vi "RANGE Startup File.vi"(11 "appended path":path) -> (3 "new file path (Not A Path if cancelled)":path)   [LabVIEW 2023]
uses:
  Drivers/Omega FMA-1600A Series Gas Flow Meter/Type Definitions/FMA1600A Gas Type.ctl
  Drivers/Omega FMA-1600A Series Gas Flow Meter/Type Definitions/FMA1600A Meter Accuracy Options.ctl
  <vilib>/Utility/file.llb/Write To Spreadsheet File (string).vi
panel:
  in  "Disable All Meters":bool
  in  "Complete":bool
  in  "Meter Accuracy Option 6":T1
  in  "Gas Meter 6":T2
  in  "Meter Accuracy Option 5":T1
  in  "Gas Meter 5":T2
  in  "Meter Accuracy Option 4":T1
  in  "Gas Meter 4":T2
  in  "Meter Accuracy Option 3":T1
  in  "Gas Meter 3":T2
  in  "Meter Accuracy Option 2":T1
  in  "Gas Meter 2":T2
  in  "Meter Accuracy Option 1":T1
  in  "Gas Meter 1":T2
  in  "Update Gas Type":bool
  in  "Tab Control":enum32{"Page 1"}(tab)
  out "Start Up File 2":string[][](array[string])
  in  "Start Up File":string[][](array[string])
  # "+/- 0.8% RDG + 0.2% FS = Standard\n+/- 0.4% RDG + 0.2% FS = HCAL (Optional when Purchased)"
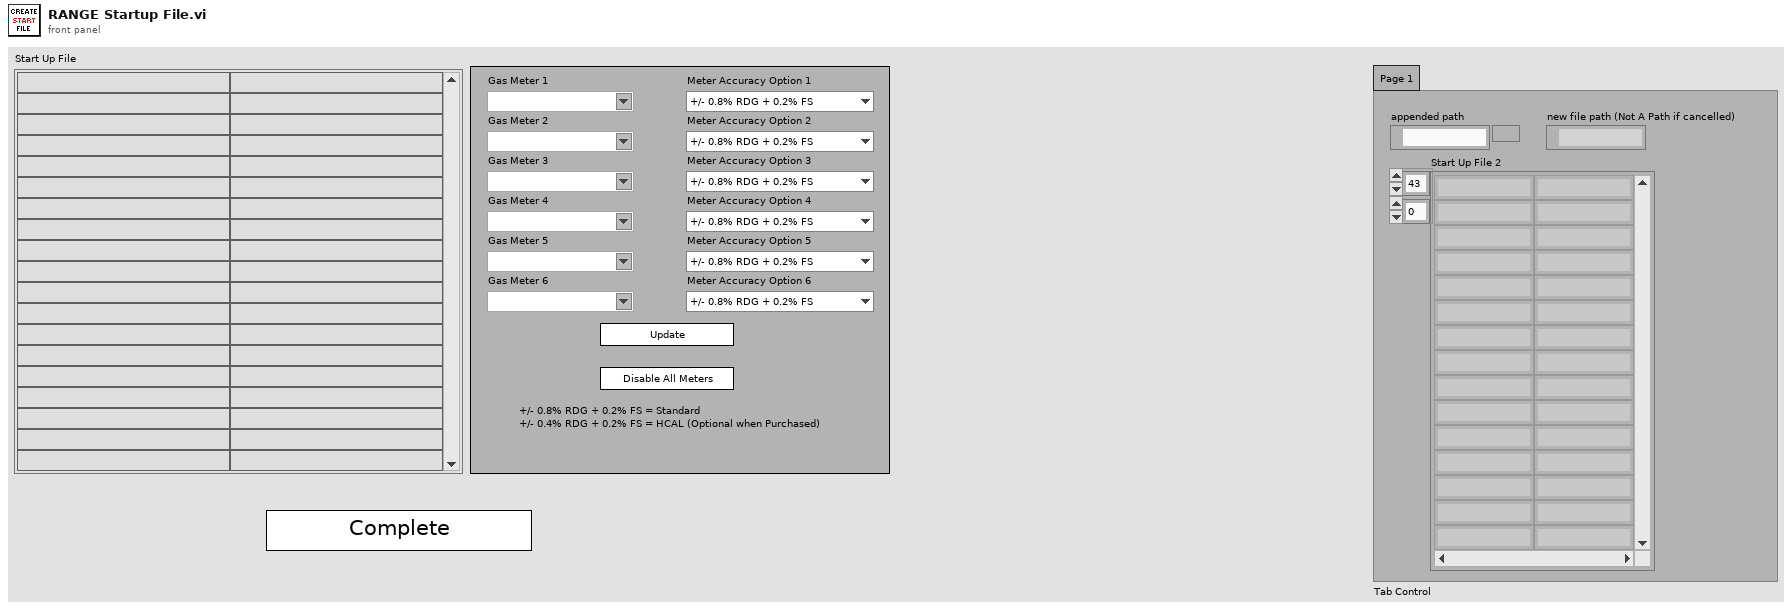
[diagram p1: front panel]
types:
  T1 = typedef "FMA1600A Meter Accuracy Options.ctl" = enum16{"+/- 0.8% RDG + 0.2% FS", "+/- 0.4% RDG + 0.2% FS"}
  T2 = typedef "FMA1600A Gas Type.ctl" = string
  T3 = enum32{"invalid app kind", "Development System", "Run Time System", "Student Edition", "Embedded LabVIEW", "Evaluation", "Custom"}
  T4 = enum32{"Invalid", "Standard", "Closed", "Hidden", "Minimized", "Maximized"}
  T5 = cluster{"Core":cluster{"Current VI Reference":refnum<vi>, "Close Panel on Exit?":bool}, "Start Up File":string[][]}
  T6 = cluster{"Current VI Reference":refnum<vi>, "Close Panel on Exit?":bool}
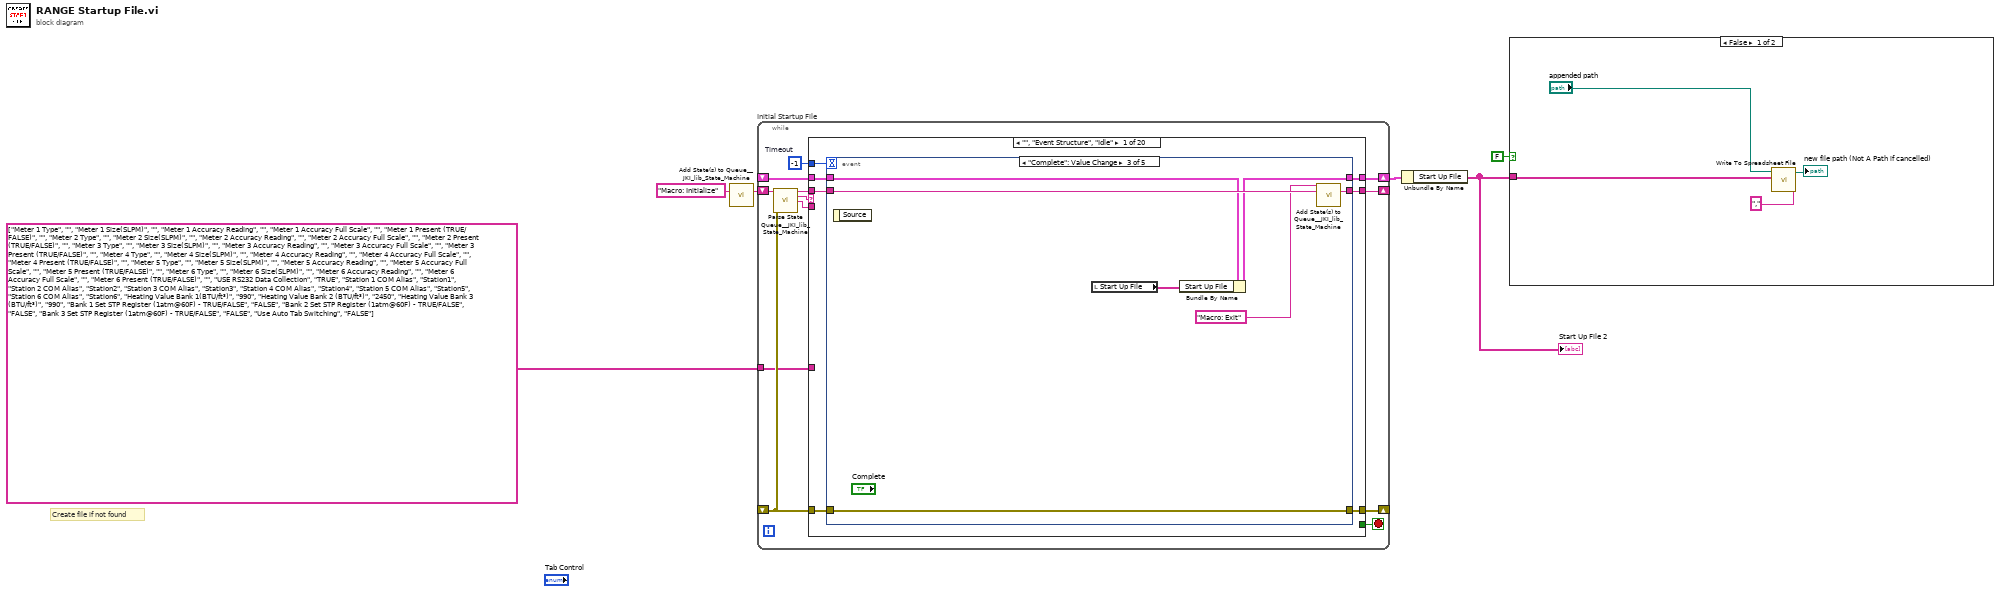
[diagram p0: block diagram]
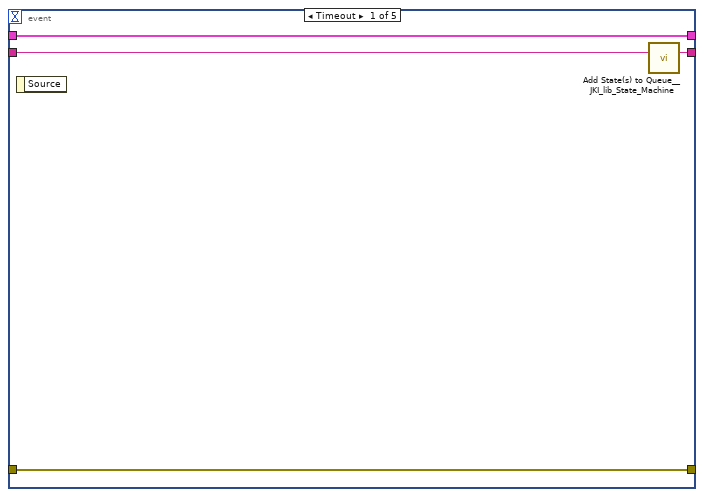
[diagram p2: hidden frame]
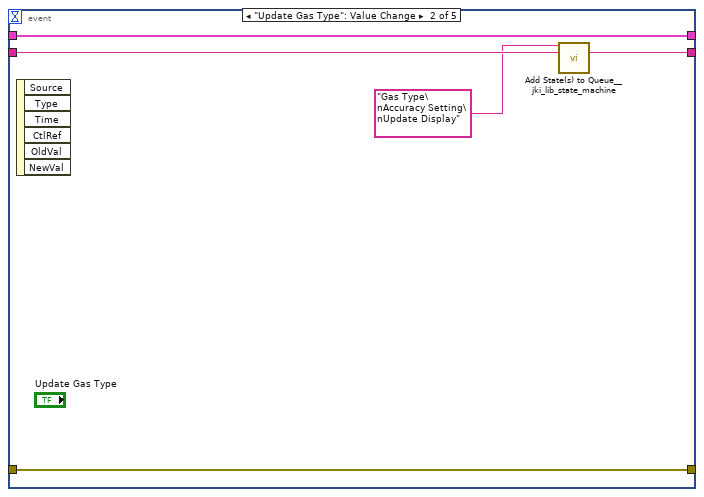
[diagram p3: hidden frame]
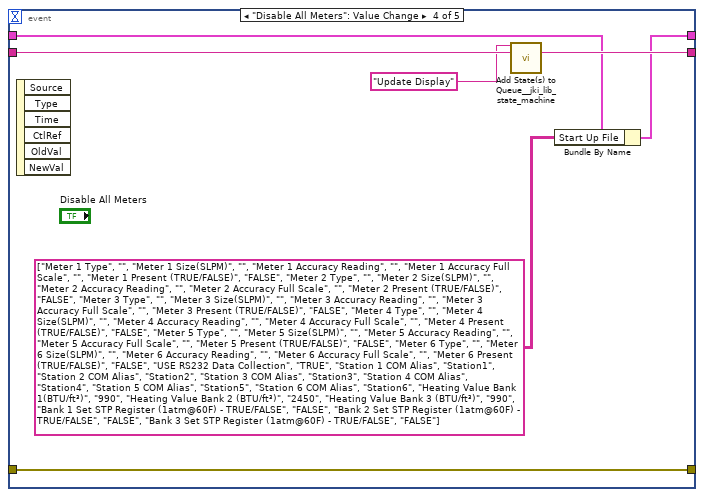
[diagram p4: hidden frame]
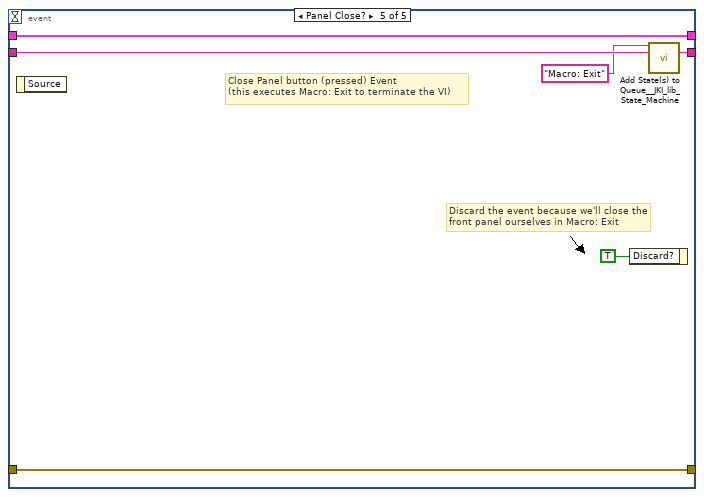
[diagram p5: hidden frame]
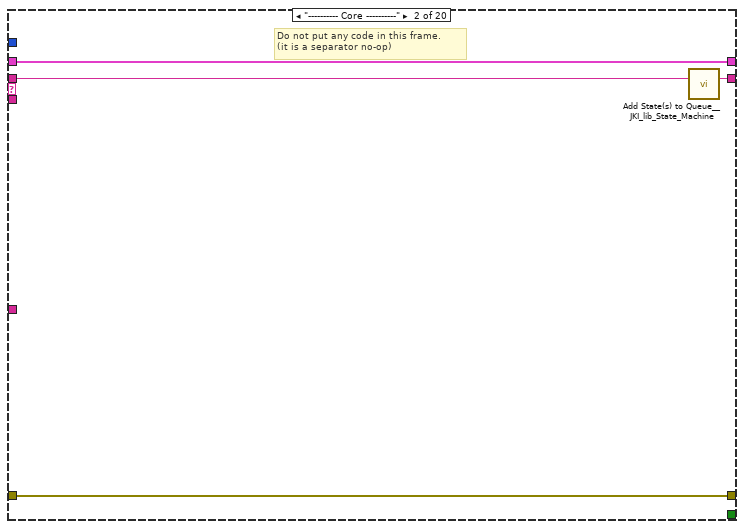
[diagram p6: hidden frame]
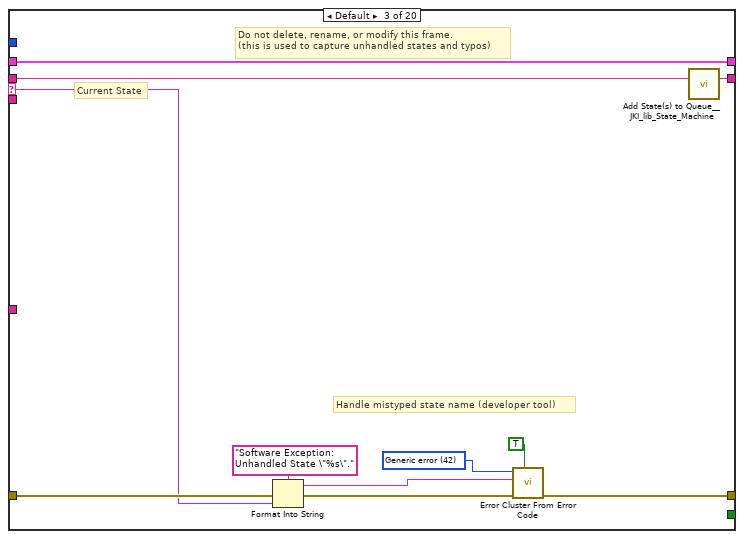
[diagram p7: hidden frame]
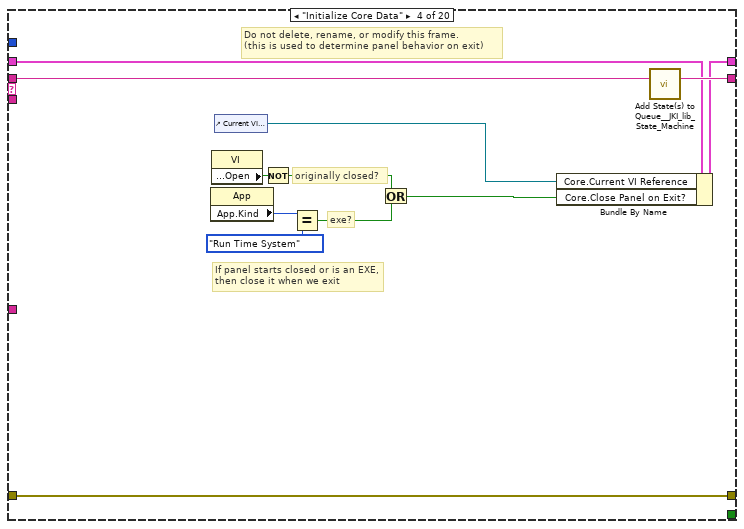
[diagram p8: hidden frame]
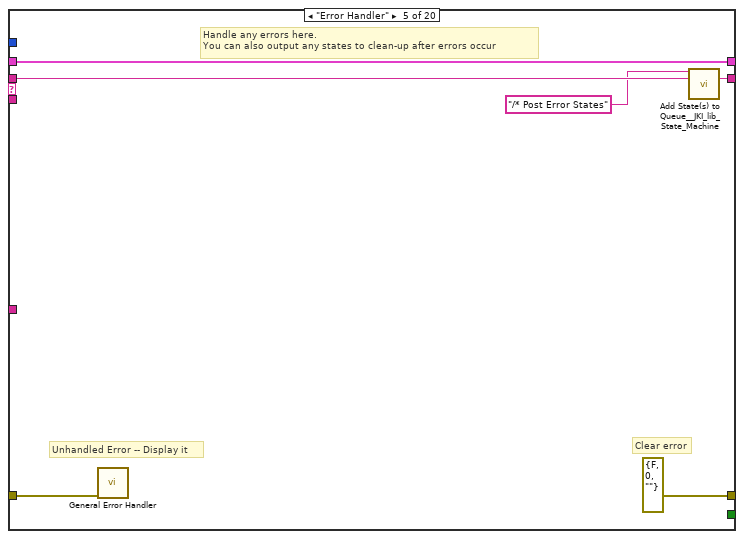
[diagram p9: hidden frame]
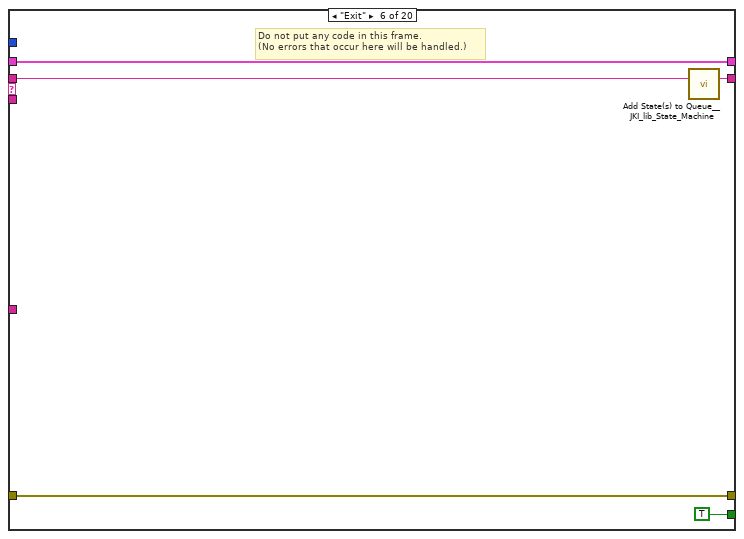
[diagram p10: hidden frame]
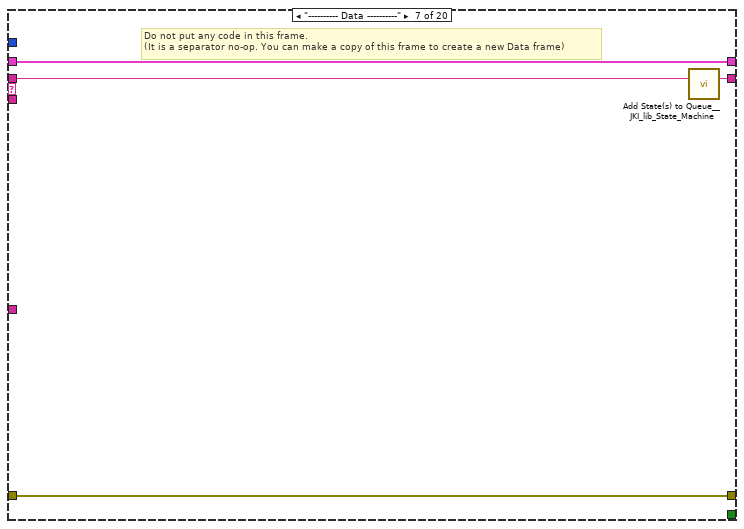
[diagram p11: hidden frame]
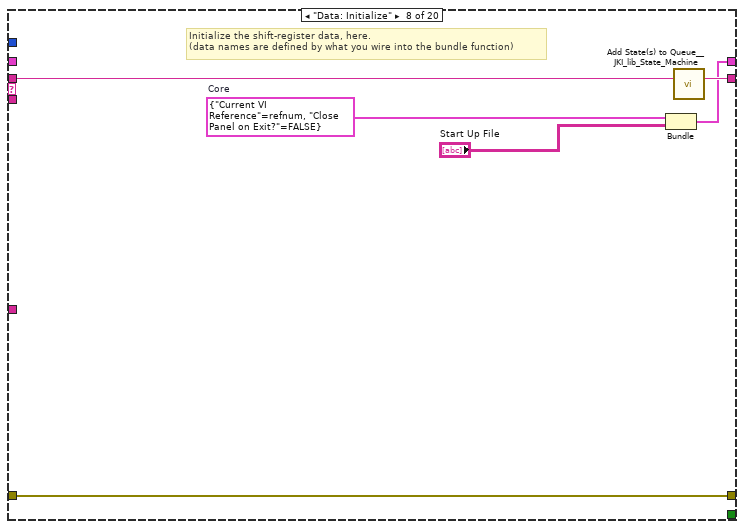
[diagram p12: hidden frame]
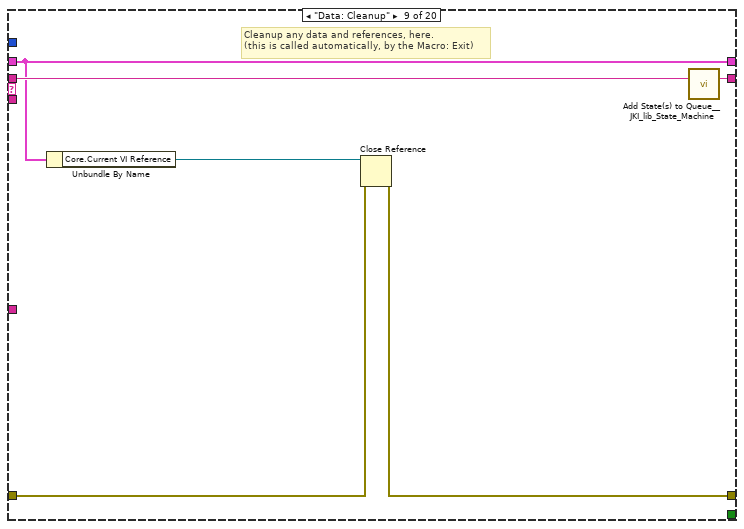
[diagram p13: hidden frame]
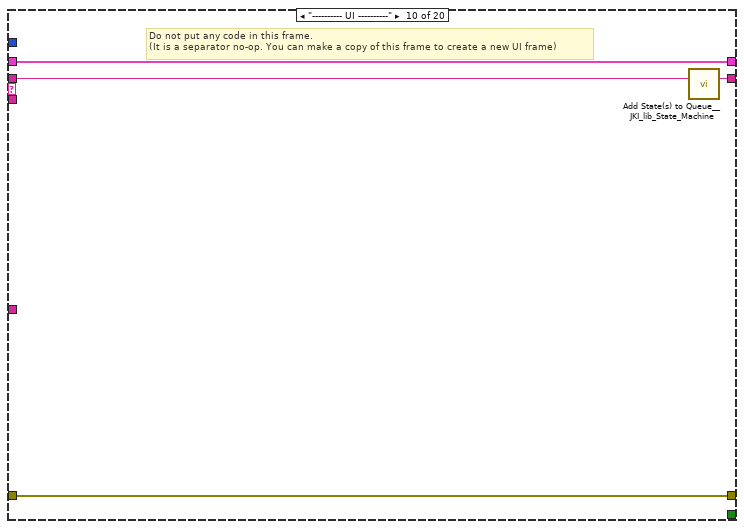
[diagram p14: hidden frame]
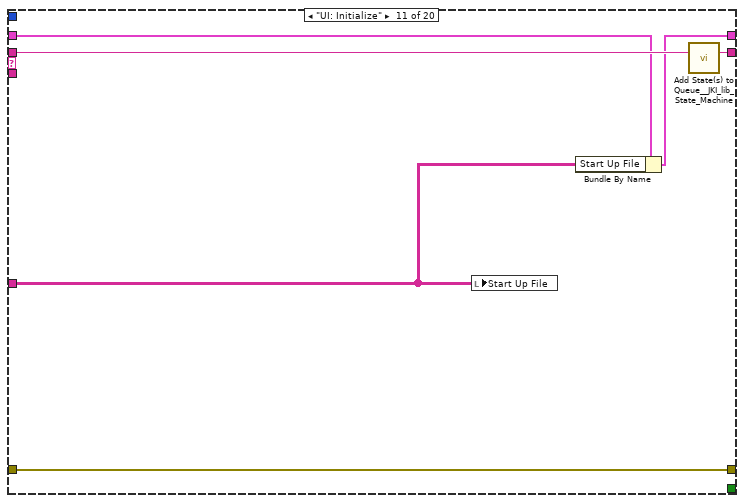
[diagram p15: hidden frame]
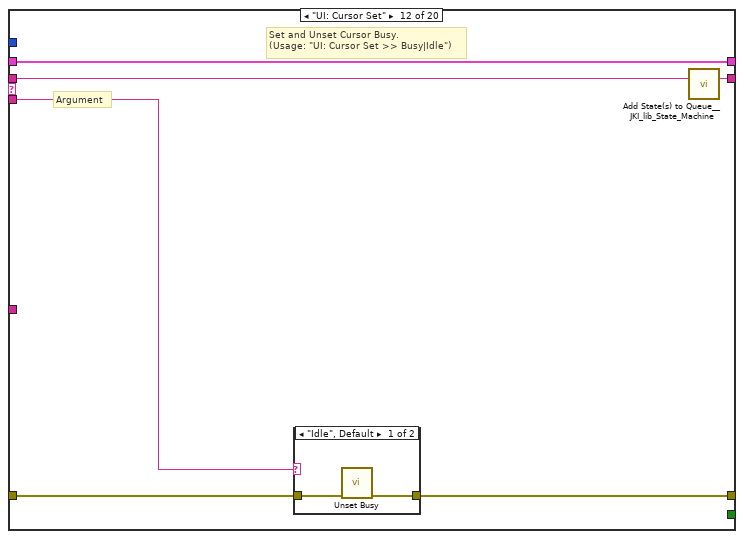
[diagram p16: hidden frame]
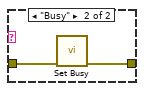
[diagram p17: hidden frame]
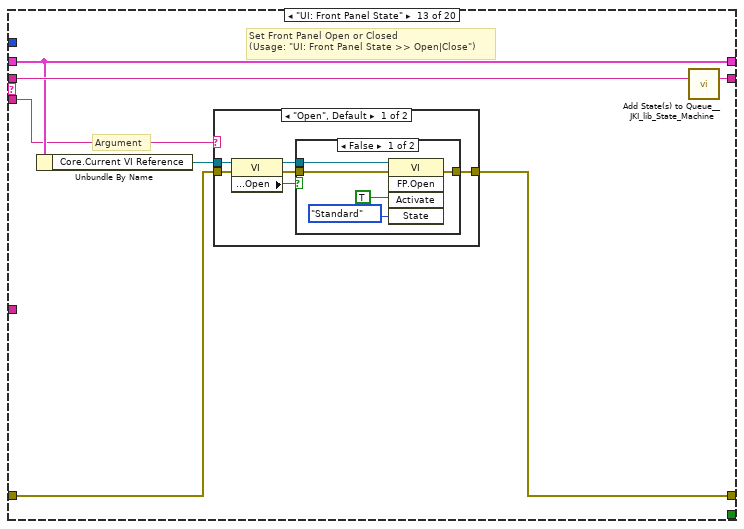
[diagram p18: hidden frame]
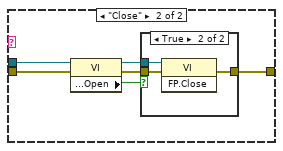
[diagram p20: hidden frame]
diagram:
  # "Create file if not found"
  n1 = call <vilib>:"Add State(s) to Queue__JKI_lib_State_Machine.vi"("State(s) in (\"\")"="Macro: Initialize") -> ("States Out"=w5:string)  [unwired: 14 in]
  n2 = while "Initial Startup File" {
    shift-right: [w11] -> w3
    shift-left: _ -> [w10]
    shift-right: [w14] -> _
    shift-left: _ -> [w8]
    shift-right: [w13] -> _
    shift-left: w5 -> [w15]
    tunnel: string[][] [["Meter 1 Type", ""], ["Meter 1 Size(SLPM)", ""], ["Meter 1 Accuracy Reading", ""], ["Meter 1 Accuracy Full Scale", ""], ["Meter 1 Present (TRUE/FALSE)", ""], ["Meter 2 Type", ""], ["Meter 2 Size(SLPM)", ""], ["Meter 2 Accuracy Reading", ""], ["Meter 2 Accuracy Full Scale", ""], ["Meter 2 Present (TRUE/FALSE)", ""], ["Meter 3 Type", ""], ["Meter 3 Size(SLPM)", ""], ["Meter 3 Accuracy Reading", ""], ["Meter 3 Accuracy Full Scale", ""], ["Meter 3 Present (TRUE/FALSE)", ""], ["Meter 4 Type", ""], ["Meter 4 Size(SLPM)", ""], ["Meter 4 Accuracy Reading", ""], ["Meter 4 Accuracy Full Scale", ""], ["Meter 4 Present (TRUE/FALSE)", ""], ["Meter 5 Type", ""], ["Meter 5 Size(SLPM)", ""], ["Meter 5 Accuracy Reading", ""], ["Meter 5 Accuracy Full Scale", ""], ["Meter 5 Present (TRUE/FALSE)", ""], ["Meter 6 Type", ""], ["Meter 6 Size(SLPM)", ""], ["Meter 6 Accuracy Reading", ""], ["Meter 6 Accuracy Full Scale", ""], ["Meter 6 Present (TRUE/FALSE)", ""], ["USE RS232 Data Collection", "TRUE"], ["Station 1 COM Alias", "Station1"], ["Station 2 COM Alias", "Station2"], ["Station 3 COM Alias", "Station3"], ["Station 4 COM Alias", "Station4"], ["Station 5 COM Alias", "Station5"], ["Station 6 COM Alias", "Station6"], ["Heating Value Bank 1(BTU/ft³)", "990"], ["Heating Value Bank 2 (BTU/ft³)", "2450"], ["Heating Value Bank 3 (BTU/ft³)", "990"], ["Bank 1 Set STP Register (1atm@60F) - TRUE/FALSE", "FALSE"], ["Bank 2 Set STP Register (1atm@60F) - TRUE/FALSE", "FALSE"], ["Bank 3 Set STP Register (1atm@60F) - TRUE/FALSE", "FALSE"], ["Use Auto Tab Switching", "FALSE"]] ("all rows 2") -> [w7]
    stop <- w12 stop-if-true
    w9 = -1  # Timeout
    n3 = call <vilib>:"Parse State Queue__JKI_lib_State_Machine.vi"("State Queue"=w15, "Error In (no error)"=w8) -> ("Remaining States"=w17:string, "Current State"=w18:string, "Arguments"=w16:string)  [unwired: 11 in]
    n4 = case shown="\"\", \"Event Structure\", \"Idle\"" w18 {
      selector: w18 -> [_ _ w59 _ _ _ _ _ _ _ _ _ _ _ _ _ _ _ _ _]
      tunnel: w17 -> [w25 w58 w63 w81 w87 w92 w96 w102 w108 w112 w118 w124 w135 w161 w166 w176 w180 w194 w208 w213]
      tunnel: w16 -> [_ _ _ _ _ _ _ _ _ _ _ w119 w129 _ _ _ _ _ _ _]
      tunnel: w10 -> [w23 w55 w61 w72 w84 w90 w93 _ w103 w109 w115 w122 w131 w158 w163 w173 w177 w192 w205 w210]
      tunnel: [w22 w56 w65 w78 errorcluster {"status"=FALSE, "code"=0, "source"=""} ("error out") w89 w94 w99 w104 w110 w116 w120 w132 w159 w164 w174 w178 w181 w201 w211] -> w14
      tunnel: w8 -> [w21 w56 w64 w78 w83 w89 w94 w99 w105 w110 w116 w121 w133 w159 w164 w174 w178 w182 w202 w211]
      tunnel: [w24 w57 w62 w80 w86 w91 w95 w101 w107 w111 w117 w123 w134 w160 w165 w175 w179 w193 w207 w212] -> w13
      tunnel: [_ _ _ _ _ TRUE _ _ _ _ _ _ _ _ _ _ _ _ _ _] -> w12
      tunnel: [w20 w55 w61 w79 w84 w90 w93 w100 w103 w109 w114 w122 w131 w158 w163 w173 w177 w191 w204 w210] -> w11
      tunnel: w9 -> [w19 _ _ _ _ _ _ _ _ _ _ _ _ _ _ _ _ _ _ _]
      tunnel: w7 -> [_ _ _ _ _ _ _ _ _ _ w113 _ _ _ _ _ _ _ _ _]
      frame "", "Event Structure", "Idle" {
        n5 = event shown="[2] \"Complete\": Value Change" {
          selector: _ -> [_ _ _ _ _]
          dyn-events: _ -> [_ _ _ _ _]
          timeout: w19 -> [_ _ _ _ _]
          tunnel: w25 -> [w29 w32 w41 w47 w54]
          tunnel: [w28 w31 w40 w46 w53] -> w24
          tunnel: w23 -> [w26 w33 w37 w44 w51]
          tunnel: [w27 w34 w39 w48 w52] -> w22
          tunnel: w21 -> [w27 w34 w39 w48 w52]
          tunnel: [w26 w33 w36 w43 w51] -> w20
          event Timeout {
            n6 = event-data() -> ()  [unwired: 1 in, 1 out]
            n7 = call <vilib>:"Add State(s) to Queue__JKI_lib_State_Machine.vi"("State(s) in (\"\")"=w29) -> ("States Out"=w28:string)  [unwired: 14 in]
          }
          event "Update Gas Type": Value Change {
            n8 = event-data() -> ()  [unwired: 1 in, 6 out]
            n9 = call <vilib>:"Add State(s) to Queue__jki_lib_state_machine.vi"("State(s) in Front (\"\")"="Gas Type\nAccuracy Setting\nUpdate Display" ("State(s) in Front (\"\")"), "State(s) in (\"\")"=w32) -> ("States Out"=w31:string)  [unwired: 13 in]
          }
          event "Complete": Value Change {
            n10 = event-data() -> ()  [unwired: 1 in, 1 out]
            n11 = local read "Start Up File"() -> (w35:string[][])
            n12 = Bundle By Name(cluster=w37, "Start Up File"=w35) -> (w36:T5)
            n13 = call <vilib>:"Add State(s) to Queue__JKI_lib_State_Machine.vi"("State(s) in Front (\"\")"="Macro: Exit", "State(s) in (\"\")"=w41) -> ("States Out"=w40:string)  [unwired: 13 in]
          }
          event "Disable All Meters": Value Change {
            n14 = event-data() -> ()  [unwired: 1 in, 6 out]
            n15 = call <vilib>:"Add State(s) to Queue__jki_lib_state_machine.vi"("State(s) in Front (\"\")"="Update Display" ("State(s) in Front (\"\")"), "State(s) in (\"\")"=w47) -> ("States Out"=w46:string)  [unwired: 13 in]
            n16 = Bundle By Name(cluster=w44, "Start Up File"=string[][] [["Meter 1 Type", ""], ["Meter 1 Size(SLPM)", ""], ["Meter 1 Accuracy Reading", ""], ["Meter 1 Accuracy Full Scale", ""], ["Meter 1 Present (TRUE/FALSE)", "FALSE"], ["Meter 2 Type", ""], ["Meter 2 Size(SLPM)", ""], ["Meter 2 Accuracy Reading", ""], ["Meter 2 Accuracy Full Scale", ""], ["Meter 2 Present (TRUE/FALSE)", "FALSE"], ["Meter 3 Type", ""], ["Meter 3 Size(SLPM)", ""], ["Meter 3 Accuracy Reading", ""], ["Meter 3 Accuracy Full Scale", ""], ["Meter 3 Present (TRUE/FALSE)", "FALSE"], ["Meter 4 Type", ""], ["Meter 4 Size(SLPM)", ""], ["Meter 4 Accuracy Reading", ""], ["Meter 4 Accuracy Full Scale", ""], ["Meter 4 Present (TRUE/FALSE)", "FALSE"], ["Meter 5 Type", ""], ["Meter 5 Size(SLPM)", ""], ["Meter 5 Accuracy Reading", ""], ["Meter 5 Accuracy Full Scale", ""], ["Meter 5 Present (TRUE/FALSE)", "FALSE"], ["Meter 6 Type", ""], ["Meter 6 Size(SLPM)", ""], ["Meter 6 Accuracy Reading", ""], ["Meter 6 Accuracy Full Scale", ""], ["Meter 6 Present (TRUE/FALSE)", "FALSE"], ["USE RS232 Data Collection", "TRUE"], ["Station 1 COM Alias", "Station1"], ["Station 2 COM Alias", "Station2"], ["Station 3 COM Alias", "Station3"], ["Station 4 COM Alias", "Station4"], ["Station 5 COM Alias", "Station5"], ["Station 6 COM Alias", "Station6"], ["Heating Value Bank 1(BTU/ft³)", "990"], ["Heating Value Bank 2 (BTU/ft³)", "2450"], ["Heating Value Bank 3 (BTU/ft³)", "990"], ["Bank 1 Set STP Register (1atm@60F) - TRUE/FALSE", "FALSE"], ["Bank 2 Set STP Register (1atm@60F) - TRUE/FALSE", "FALSE"], ["Bank 3 Set STP Register (1atm@60F) - TRUE/FALSE", "FALSE"]] ("all rows 2")) -> (w43:T5)
          }
          event Panel Close? {
            # "Discard the event because we'll close the front panel ourselves in Macro: Exit"
            # "Close Panel button (pressed) Event\n(this executes Macro: Exit to terminate the VI)"
            n17 = event-data() -> ()  [unwired: 1 in, 1 out]
            n18 = event-data("Discard?"=TRUE) -> ()  [unwired: 1 in, 1 out]
            n19 = call <vilib>:"Add State(s) to Queue__JKI_lib_State_Machine.vi"("State(s) in Front (\"\")"="Macro: Exit", "State(s) in (\"\")"=w54) -> ("States Out"=w53:string)  [unwired: 13 in]
          }
        }
      }
      frame "---------- Core ----------" {
        # "Do not put any code in this frame.\n(it is a separator no-op)"
        n20 = call <vilib>:"Add State(s) to Queue__JKI_lib_State_Machine.vi"("State(s) in (\"\")"=w58) -> ("States Out"=w57:string)  [unwired: 14 in]
      }
      frame Default {
        w68 = 42 items=["No error", "Argument error", "Memory is full", "Out of zone", "End of file", "File already open", "Generic file I/O error", "File not found", "File permission error", "Disk is full", "Duplicate path", "Too many files open", "System feature not enabled", "Resource file not found", "Cannot add resource", "Resource not found", "Image not found", "Image memory error", "Pen does not exist", "Config type invalid", "Config token not found", "Config parse error", "Config memory error", "Bad external code format", "Bad external code offset", "External code not present", "Null window", "Destroy window error", "Null menu", "Print aborted", "Bad print record", "Print driver error", "Windows error during printing", "Memory error during printing", "Print dialog error", "Generic print error", "Invalid device refnum", "Device not found", "Device parameter error", "Device unit error", "Cannot open device", "Device call aborted", "Generic error", "Cancelled by user", "Object ID too low", "Object ID too high", "Object not in heap", "Unknown heap", "Unknown object (invalid DefProc)", "Unknown object (DefProc not in table)", "Message out of range", "Invalid (null) method", "Unknown message", "Manager call not supported", "Bad address", "Network operation in progress", "Network operation timed out", "Connection is busy", "Network attribute not supported", "Network error", "Address in use", "System out of memory", "Connection aborted", "Connection refused", "Not connected", "Already connected", "Connection closed", "Initialization error (interapplication manager)", "Bad occurrence", "Wait on unbound occurrence handler", "Occurrence queue overflow", "Datalog type conflict", "Unused", "Unrecognized type (interapplication manager)", "Memory corrupt", "Failed to make temporary DLL", "Old CIN version", "Drag socket not found", "Failed to load drop-object", "Failed to register OLE object", "Failed to release OLE object", "Format specifier type mismatch", "Unknown format specifier", "Too few format specifiers", "Too many format specifiers", "Scan failed", "Newer CIN version", "Error converting to variant", "Runtime menu error", "Password tampered", "Variant attribute not found", "Incompatible variant data type", "Event data is not available", "Event Store is not present", "Occurrence is not found", "Event Queue is not created", "Event info is not available", "Refnum passed is NULL", "Error retrieving Class GUID", "Error retrieving CoClass GUID", "Error retrieving TypeLib GUID.", "Bad built application magic bytes.", "Specific driver is different from the specific driver associated with the Logical Name.", "There is no session opened to the class driver.", "Max Error", "MAX - Error with config objects", "MAX - Error loading configuration", "MAX - Group not supported"]
        # "Current State"
        # "Do not delete, rename, or modify this frame.\n(this is used to capture unhandled states and typos)"
        # "Handle mistyped state name (developer tool)"
        n21 = Format Into String(format string="Software Exception: Unhandled State \"%s\"." ("message"), error in=w64, w59) -> (resulting string=w67:string, error out=w66:errorcluster)  [unwired: 1 in]
        n22 = call <vilib>:"Error Cluster From Error Code.vi"("show call chain? (False)"=TRUE, "error in (no error)"=w66, "error message (\"\")"=w67, "error code (0)"=w68) -> ("error out"=w65:errorcluster)  [unwired: 5 in]
        n23 = call <vilib>:"Add State(s) to Queue__JKI_lib_State_Machine.vi"("State(s) in (\"\")"=w63) -> ("States Out"=w62:string)  [unwired: 14 in]
      }
      frame "Initialize Core Data" {
        # "Do not delete, rename, or modify this frame.\n(this is used to determine panel behavior on exit)"
        # "originally closed?"
        # "exe?"
        # "If panel starts closed or is an EXE, then close it when we exit"
        n24 = property class="App"() -> ("App.Kind"=w76:T3)  [unwired: 2 in, 2 out]
        n25 = property class="VI"() -> ("Front Panel.Open"=w77:bool)  [unwired: 2 in, 2 out]
        n26 = control-ref of="Current VI Reference"() -> (w70:refnum<vi>)
        n27 = Not(x=w77) -> (.not. x?=w74:bool)
        n28 = Equal?(x=w76, y=T3."Run Time System" ("Application:Kind")) -> (x = y?=w73:bool)
        n29 = Or(x=w74, y=w73) -> (x .or. y?=w71:bool)
        n30 = Bundle By Name(cluster=w72, "Core.Current VI Reference"=w70, "Core.Close Panel on Exit?"=w71) -> (w79:T5)
        n31 = call <vilib>:"Add State(s) to Queue__JKI_lib_State_Machine.vi"("State(s) in (\"\")"=w81) -> ("States Out"=w80:string)  [unwired: 14 in]
      }
      frame "Error Handler" {
        # "Unhandled Error -- Display it"
        # "Handle any errors here.\nYou can also output any states to clean-up after errors occur"
        # "Clear error"
        n32 = call <vilib>:"General Error Handler.vi"("error in (no error)"=w83) -> ()  [unwired: 10 in, 5 out]
        n33 = call <vilib>:"Add State(s) to Queue__JKI_lib_State_Machine.vi"("State(s) in Front (\"\")"="/* Post Error States", "State(s) in (\"\")"=w87) -> ("States Out"=w86:string)  [unwired: 13 in]
      }
      frame "Exit" {
        # "Do not put any code in this frame.\n(No errors that occur here will be handled.)"
        n34 = call <vilib>:"Add State(s) to Queue__JKI_lib_State_Machine.vi"("State(s) in (\"\")"=w92) -> ("States Out"=w91:string)  [unwired: 14 in]
      }
      frame "---------- Data ----------" {
        # "Do not put any code in this frame.\n(It is a separator no-op. You can make a copy of this frame to create a new Data frame)"
        n35 = call <vilib>:"Add State(s) to Queue__JKI_lib_State_Machine.vi"("State(s) in (\"\")"=w96) -> ("States Out"=w95:string)  [unwired: 14 in]
      }
      frame "Data: Initialize" {
        w98 = T6 {"Current VI Reference"=refnum, "Close Panel on Exit?"=FALSE}  # Core
        # "Initialize the shift-register data, here.\n(data names are defined by what you wire into the bundle function)"
        n36 = Bundle("Core"=w98, "Start Up File"="Start Up File") -> (w100:T5)  [unwired: 1 in]
        n37 = call <vilib>:"Add State(s) to Queue__JKI_lib_State_Machine.vi"("State(s) in (\"\")"=w102) -> ("States Out"=w101:string)  [unwired: 14 in]
      }
      frame "Data: Cleanup" {
        # "Cleanup any data and references, here.\n(this is called automatically, by the Macro: Exit)"
        n38 = Unbundle By Name(w103) -> ("Core.Current VI Reference"=w106:refnum<vi>)
        n39 = Close Reference(reference=w106, error in (no error)=w105) -> (error out=w104:errorcluster)
        n40 = call <vilib>:"Add State(s) to Queue__JKI_lib_State_Machine.vi"("State(s) in (\"\")"=w108) -> ("States Out"=w107:string)  [unwired: 14 in]
      }
      frame "---------- UI ----------" {
        # "Do not put any code in this frame.\n(It is a separator no-op. You can make a copy of this frame to create a new UI frame)"
        n41 = call <vilib>:"Add State(s) to Queue__JKI_lib_State_Machine.vi"("State(s) in (\"\")"=w112) -> ("States Out"=w111:string)  [unwired: 14 in]
      }
      frame "UI: Initialize" {
        n42 = local write "Start Up File"(w113) -> ()
        n43 = Bundle By Name(cluster=w115, "Start Up File"=w113) -> (w114:T5)
        n44 = call <vilib>:"Add State(s) to Queue__JKI_lib_State_Machine.vi"("State(s) in (\"\")"=w118) -> ("States Out"=w117:string)  [unwired: 14 in]
      }
      frame "UI: Cursor Set" {
        # "Argument"
        # "Set and Unset Cursor Busy.\n(Usage: \"UI: Cursor Set >> Busy|Idle\")"
        n45 = case shown="\"Idle\", Default" w119 {
          tunnel: w121 -> [w126 w128]
          tunnel: [w125 w127] -> w120
          frame "Idle", Default {
            n46 = call <vilib>:"Unset Busy.vi"("error in (no error)"=w126) -> ("error out"=w125:errorcluster)  [unwired: 10 in]
          }
          frame "Busy" {
            n47 = call <vilib>:"Set Busy.vi"("error in (no error)"=w128) -> ("error out"=w127:errorcluster)  [unwired: 9 in, 1 out]
          }
        }
        n48 = call <vilib>:"Add State(s) to Queue__JKI_lib_State_Machine.vi"("State(s) in (\"\")"=w124) -> ("States Out"=w123:string)  [unwired: 14 in]
      }
      frame "UI: Front Panel State" {
        # "Argument"
        # "Set Front Panel Open or Closed\n(Usage: \"UI: Front Panel State >> Open|Close\")"
        n49 = Unbundle By Name(w131) -> ("Core.Current VI Reference"=w130:refnum<vi>)
        n50 = case shown="\"Open\", Default" w129 {
          tunnel: w133 -> [w139 w152]
          tunnel: [w141 w153] -> w132
          tunnel: w130 -> [w140 w150]
          frame "Open", Default {
            n51 = property class="VI"(reference=w140, error in=w139) -> (reference out=w137:refnum<vi>, error out=w138:errorcluster, "Front Panel.Open"=w136:bool)
            n52 = case shown="False" w136 {
              tunnel: [w144 w147] -> w141
              tunnel: w138 -> [w143 w147]
              tunnel: w137 -> [w142 _]
              frame False {
                n53 = invoke class="VI" method="FP.Open"(reference=w142, error in=w143, "Activate"=TRUE, "State"=T4."Standard") -> (error out=w144:errorcluster)  [unwired: 1 in, 4 out]
              }
              frame True {
              }
            }
          }
          frame "Close" {
            n54 = property class="VI"(reference=w150, error in=w152) -> (reference out=w149:refnum<vi>, error out=w151:errorcluster, "Front Panel.Open"=w148:bool)
            n55 = case shown="True" w148 {
              tunnel: [w154 w157] -> w153
              tunnel: w151 -> [w154 w156]
              tunnel: w149 -> [_ w155]
              frame False {
              }
              frame True {
                n56 = invoke class="VI" method="FP.Close"(reference=w155, error in=w156) -> (error out=w157:errorcluster)  [unwired: 1 in, 2 out]
              }
            }
          }
        }
        n57 = call <vilib>:"Add State(s) to Queue__JKI_lib_State_Machine.vi"("State(s) in (\"\")"=w135) -> ("States Out"=w134:string)  [unwired: 14 in]
      }
      frame "---------- Macro ----------" {
        # "Do not put any code in this frame.\n(It is a separator no-op. You can make a copy of this frame to create a new Macro frame)"
        n58 = call <vilib>:"Add State(s) to Queue__JKI_lib_State_Machine.vi"("State(s) in (\"\")"=w161) -> ("States Out"=w160:string)  [unwired: 14 in]
      }
      frame "Macro: Initialize" {
        w162 = "Data: Initialize\nInitialize Core Data\nUI: Initialize\nUI: Front Panel State >> Open"  # Data: Initialize Initialize Core Data UI: Initialize UI: Front Panel State >> Open
        # "Initialization Macro\n(This is called once, when the VI starts)"
        n59 = call <vilib>:"Add State(s) to Queue__JKI_lib_State_Machine.vi"("State(s) in Front (\"\")"=w162, "State(s) in (\"\")"=w166) -> ("States Out"=w165:string)  [unwired: 13 in]
      }
      frame "Macro: Exit" {
        # "Exit Macro\n(This is called once, when the VI exits)"
        n60 = Unbundle By Name(w173) -> ("Core.Close Panel on Exit?"=w172:bool)
        n61 = Select(t="UI: Front Panel State >> Close", s=w172, f="") -> (s? t:f=w169:string)
        n62 = call <vilib>:"Add State(s) to Queue__JKI_lib_State_Machine.vi"("State(s) in (\"\")"=w169, "State(s) at Back (\"\")"="Data: Cleanup\nExit") -> ("States Out"=w167:string)  [unwired: 13 in]
        n63 = call <vilib>:"Add State(s) to Queue__JKI_lib_State_Machine.vi"("State(s) in Front (\"\")"=w167, "State(s) in (\"\")"=w176) -> ("States Out"=w175:string)  [unwired: 13 in]
      }
      frame "---------- New Category ----------" {
        # "Template Separator\n(You can make a copy of, or modify, this frame)"
        n64 = call <vilib>:"Add State(s) to Queue__JKI_lib_State_Machine.vi"("State(s) in (\"\")"=w180) -> ("States Out"=w179:string)  [unwired: 14 in]
      }
      frame "Gas Type" {
        n65 = Unbundle By Name(w192) -> ("Start Up File"=w189:string[][])
        n66 = property on="Gas Meter 1" class="CmbBox (strict)"() -> ("Text.Text"=w188:string)  [unwired: 2 in, 2 out]
        n67 = property on="Gas Meter 2" class="CmbBox (strict)"() -> ("Text.Text"=w187:string)  [unwired: 2 in, 2 out]
        n68 = property on="Gas Meter 3" class="CmbBox (strict)"() -> ("Text.Text"=w186:string)  [unwired: 2 in, 2 out]
        n69 = property on="Gas Meter 4" class="CmbBox (strict)"() -> ("Text.Text"=w185:string)  [unwired: 2 in, 2 out]
        n70 = property on="Gas Meter 5" class="CmbBox (strict)"() -> ("Text.Text"=w184:string)  [unwired: 2 in, 2 out]
        n71 = property on="Gas Meter 6" class="CmbBox (strict)"() -> ("Text.Text"=w183:string)  [unwired: 2 in, 2 out]
        n72 = call "RANGE Update Meter Types.vi"("Start Up File in"=w189, "Meter Type 1"=w188, "Meter Type 2"=w187, "Meter Type 3"=w186, "Meter Type 4"=w185, "Error In"=w182, "Meter Type 5"=w184, "Meter Type 6"=w183) -> ("Start Up File out"=w190:string[][], "Error Out"=w181:errorcluster)  [unwired: 10 in]
        n73 = Bundle By Name(cluster=w192, "Start Up File"=w190) -> (w191:T5)
        n74 = call <vilib>:"Add State(s) to Queue__JKI_lib_State_Machine.vi"("State(s) in (\"\")"=w194) -> ("States Out"=w193:string)  [unwired: 14 in]
      }
      frame "Accuracy Setting" {
        n75 = Unbundle By Name(w205) -> ("Start Up File"=w206:string[][])
        n76 = call "RANGE Update Accuracy Settings.vi"("Start Up File in"=w206, "Meter Accuracy Option 1"="Meter Accuracy Option 1", "Meter Accuracy Option 2"="Meter Accuracy Option 2", "Meter Accuracy Option 3"="Meter Accuracy Option 3", "Meter Accuracy Option 4"="Meter Accuracy Option 4", "Error In"=w202, "Meter Accuracy Option 5"="Meter Accuracy Option 5", "Meter Accuracy Option 6"="Meter Accuracy Option 6") -> ("Start Up File out"=w203:string[][], "Error Out"=w201:errorcluster)  [unwired: 10 in]
        n77 = Bundle By Name(cluster=w205, "Start Up File"=w203) -> (w204:T5)
        n78 = call <vilib>:"Add State(s) to Queue__JKI_lib_State_Machine.vi"("State(s) in (\"\")"=w208) -> ("States Out"=w207:string)  [unwired: 14 in]
      }
      frame "Update Display" {
        n79 = Unbundle By Name(w210) -> ("Start Up File"=w209:string[][])
        n80 = local write "Start Up File"(w209) -> ()
        n81 = call <vilib>:"Add State(s) to Queue__JKI_lib_State_Machine.vi"("State(s) in (\"\")"=w213) -> ("States Out"=w212:string)  [unwired: 14 in]
      }
    }
  }
  n82 = Unbundle By Name(w3) -> ("Start Up File"=w2:string[][])
  "Start Up File 2" <- w2
  n83 = case shown="False" FALSE {
    tunnel: w2 -> [w216 _]
    frame False {
      n84 = call-poly <vilib>:"Write To Spreadsheet File.vi"("delimiter (\\t)"="," ("delimiter (\\t)"), "2D data"=w216, "file path (dialog if empty)"="appended path") -> ("new file path (Not A Path if cancelled)"=→"new file path (Not A Path if cancelled)":path)  [unwired: 5 in]
    }
    frame True {
    }
  }
